vi "process_exit_callback.vi"(4 "ProcessExit event":refnum<user-event>, 5 "Event Data":cluster{"sender":refnum<k24>, "e":refnum<k24>}, 6 "Control Ref":refnum<k24>, 7 "Event Common Data":T1) -> ()   [LabVIEW 2021, in "JKI dotNET System Exec.lvlib" / "dotnet_system_exec.lvclass"]
doc: "Process Exit Callback VI\n\n-----------------------------------------------\nJKI .NET System Exec 1.0.0.6\nJavier Ruiz - JKI\nCopyright (c) 2021, JKI\njki.net"
uses:
  dotnet_system_exec.lvclass
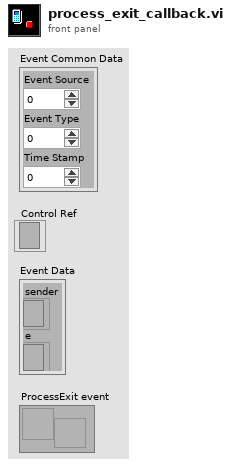
[diagram p1: front panel]
types:
  T1 = cluster{"Event Source":i32, "Event Type":u32, "Time Stamp":u32}
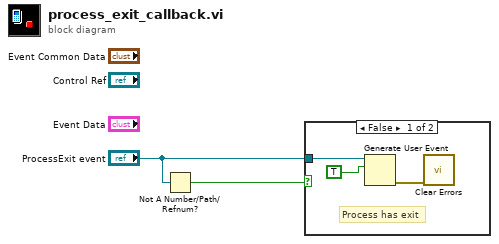
[diagram p0: block diagram]
diagram:
  n1 = Not A Number/Path/Refnum?(number/path/refnum="ProcessExit event") -> (NaN/Path/Refnum?=w2:bool)
  n2 = case shown="False" w2 {
    tunnel: "ProcessExit event" -> [w5 _]
    frame False {
      # "Process has exit"
      n3 = Generate User Event(user event=w5, event data cluster=TRUE ("event data")) -> (error out=w4:errorcluster)  [unwired: 2 in, 1 out]
      n4 = call <vilib>:"Clear Errors.vi"("error in (no error)"=w4) -> ()  [unwired: 5 in, 2 out]
    }
    frame True {
    }
  }
